vi "SVPO RMS Level (N Ch DBL Array).vi"(6 "restart averaging? (F)":bool, 10 "sampling rate [Hz]":dbl=1.0, 11 "scaled signals [EU]":dbl[][](array[numeric])) -> (3 "RMS levels":dbl[](array[numeric]), 4 "durations [s]":dbl[](array[numeric]))   [LabVIEW 2017, in "SoundVib_VibrationLevel.lvlib"]
doc: "Computes the root-mean-square (RMS) level of scaled time waveform signals and scaled array signals. <B>scaled signal [EU]</B> should have a zero DC component. You can attenuate the DC component with hardware AC-coupling filters and with software high-pass filters. Use this VI on embedded targets that have limited computational resources. Wire data to the <B>scaled signal [EU]</B> input to determine the polymorphic instance to use or manually select the instance."
uses:
  <vilib>/addons/Sound and Vibration/svt_Level/SoundVib_VibrationLevel.lvlib
  <vilib>/addons/_NISVFA/_Shared subVIs/Controls/svc_RMS Level State.ctl
  <vilib>/Analysis/baseanly.llb/Dot Product.vi
  <vilib>/Analysis/baseanly.llb/Real Dot Product.vi
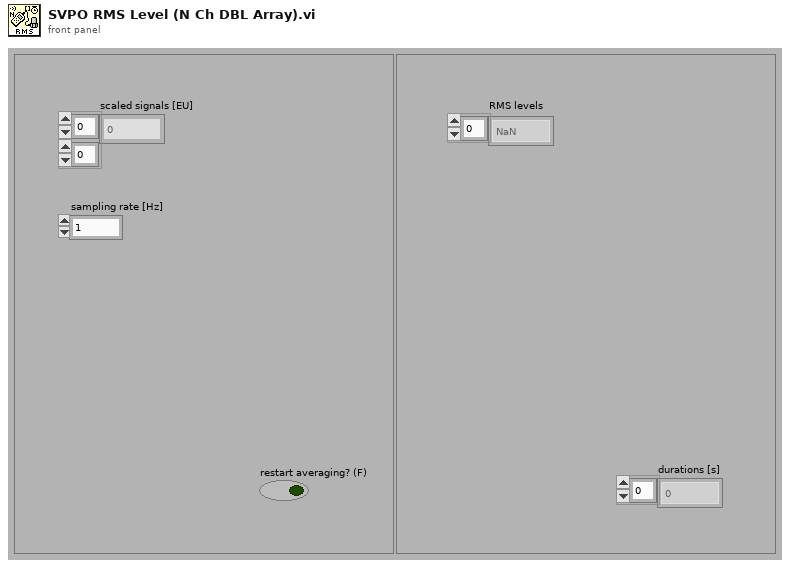
[diagram p1: front panel]
types:
  T1 = typedef "svc_RMS Level State.ctl" = cluster{"Squared Sum":dbl, "Size":u64, "timestamp":timestamp}
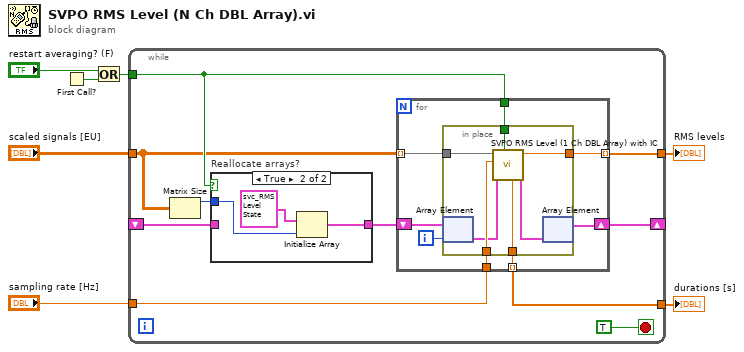
[diagram p0: block diagram]
diagram:
  n1 = First Call?() -> (First Call?: T/F=w7:bool)
  n2 = Or(x="restart averaging? (F)", y=w7) -> (x .or. y?=w5:bool)
  n3 = while {
    tunnel: w5 -> [w10]
    tunnel: "scaled signals [EU]" -> [w9]
    shift-right: [w16] -> _
    shift-left: _ -> [w15]
    tunnel: [w13] -> w3
    tunnel: [w12] -> w2
    tunnel: "sampling rate [Hz]" -> [w11]
    stop <- TRUE stop-if-true
    n4 = Matrix Size(0:w9) -> (1:w8:i32)  [unwired: 1 out]
    n5 = case "Reallocate arrays?" shown="True" w10 {
      tunnel: [w18 w21] -> w14
      tunnel: w15 -> [w18 _]
      tunnel: w8 -> [_ w19]
      frame False {
      }
      frame True {
        n6 = Initialize Array(T1 {"Squared Sum"=0.0, "Size"=0, "timestamp"=timestamp(0 s since 1904-01-01)} ("Final Conditions"), w19) -> (w21:T1[])
      }
    }
    n7 = for {
      tunnel: w9 -> [w29] mode=indexing
      tunnel: [w28] -> w13 mode=indexing
      tunnel: w10 -> [w27]
      tunnel: [w26] -> w12 mode=indexing
      tunnel: w11 -> [w25]
      shift-right: [w22] -> w16
      shift-left: w14 -> [w24]
      i -> [w23]
      n8 = in-place {
        in-place-border: w29 -> [w36]
        in-place-border: [w35] -> w28
        in-place-border: w27 -> [w34]
        in-place-border: [w33] -> w26
        in-place-border: w25 -> [w32]
        n9 = in-place-array #1(w24, w23) -> (w31:T1)
        n10 = call <vilib>:"SVPO RMS Level (1 Ch DBL Array) with IC.vi"("restart averaging? (F)"=w34, "initial conditions"=w31, "sampling rate [Hz]"=w32, "scaled signal [EU]"=w36) -> ("final conditions"=w30:T1, "RMS level"=w35:dbl, "duration [s]"=w33:dbl)  [unwired: 5 in]
        n11 = in-place-array #1(w30) -> (w22:T1[])  [unwired: 1 out]
      }
    }
  }
  "RMS levels" <- w3
  "durations [s]" <- w2
